vi "Enable List Mode.vi"(8 "error in (no error)":errorcluster, 10 "Enable List Mode (F: False)":bool, 11 "VISA resource name":refnum<visa-resource-name>) -> (0 "error out":errorcluster, 3 "VISA resource name out":refnum<visa-resource-name>)   [LabVIEW 2022 SP3, in "BK Precision 911X Series.lvlib"]
doc: "Enables or disables list mode. Configure all list parameters first prior to enabling list mode. To run a list, send a trigger after running this vi.\n\n<b>Note: List program functionality is not available on model 9117.</b>"
uses:
  <instrlib>/BK Precision 911X Series/BK Precision 911X Series.lvlib
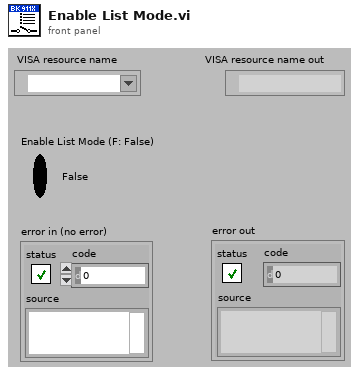
[diagram p1: front panel]
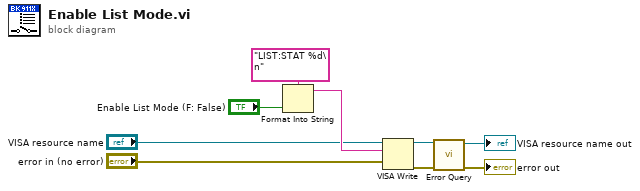
[diagram p0: block diagram]
diagram:
  n1 = Format Into String(format string="LIST:STAT %d\n", "Enable List Mode (F: False)") -> (resulting string=w5:string)  [unwired: 2 in, 1 out]
  n2 = VISA Write(VISA resource name="VISA resource name", write buffer=w5, error in (no error)="error in (no error)") -> (VISA resource name out=w4:refnum<visa-resource-name>, error out=w3:errorcluster)  [unwired: 1 out]
  n3 = call <instrlib>:"Error Query.vi"("error in (no error)"=w3, "VISA resource name"=w4) -> ("error out"=→"error out":errorcluster, "VISA resource name out"=→"VISA resource name out":refnum<visa-resource-name>)  [unwired: 6 in, 2 out]
